vi "Impedance_Multi_WrapSingle.vi"() -> ()   [LabVIEW 2021]
uses:
  <vilib>/Analysis/1siggen.llb/Ramp Pattern by Samples.vi
  <vilib>/Analysis/baseanly.llb/Mean (DBL).vi
  <vilib>/Analysis/NI_AALBase.lvlib
panel:
  out "Test Number":i32
  in  "Num Avg":i32=5
  out "Mean Phase":dbl format="%0.2f"
  out "Mean Mag":dbl format="%.4p"
  out "Phase Graph":cluster{dbl[], "Ramp Pattern":dbl[]}(graph)
  in  "amplitude":dbl=0.1 format="%0.2p"
  in  "SampRate":dbl=250000.0 format="%0.2f"
  in  "Test Time":dbl=1.0 format="%#_6p"
  out "Mag Graph":cluster{dbl[], "Ramp Pattern":dbl[]}(graph)
  in  "samples":i32=128
  in  "start":dbl format="%#.4p"
  in  "end freq":dbl=1.0 format="%#.4p"
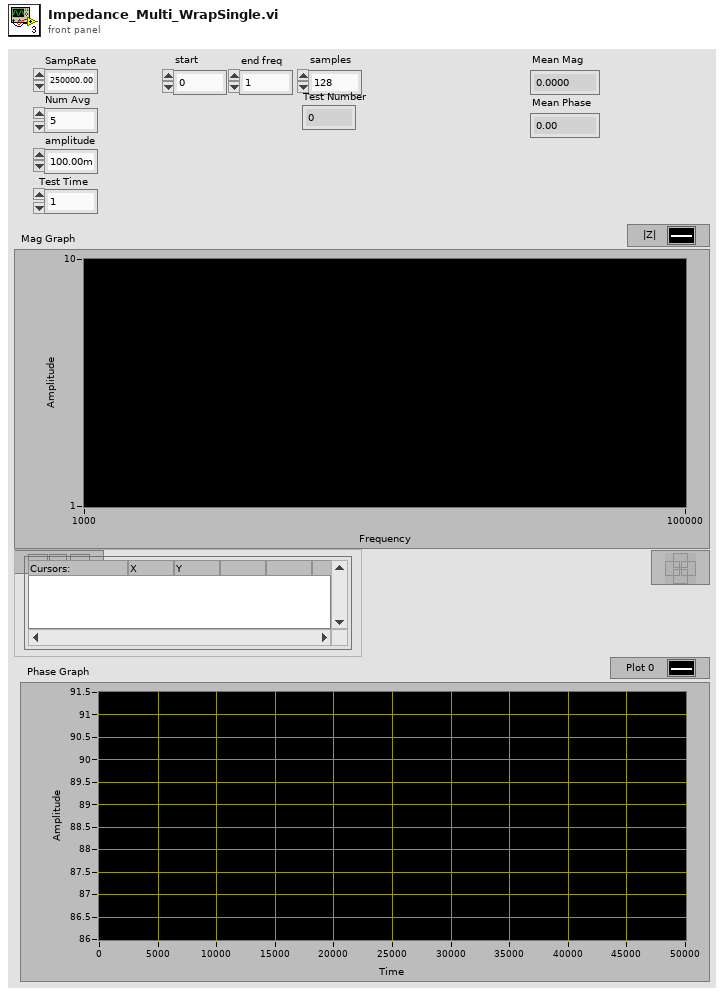
[diagram p1: front panel]
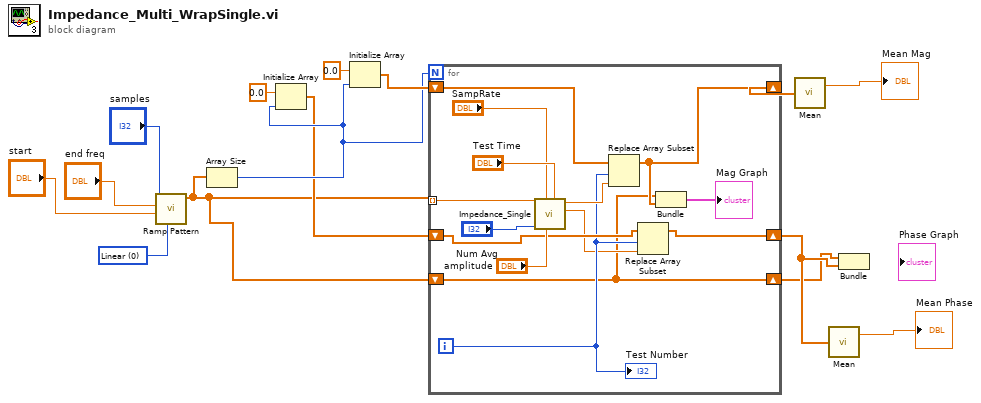
[diagram p0: block diagram]
diagram:
  w12 = u16 0 items=["Linear", "Logarithmic"] ("type")
  n1 = call-poly <vilib>:"Ramp Pattern.vi"("type"=w12, "start"="start", "end"="end freq", "samples"="samples") -> ("Ramp Pattern"=w3:dbl[])  [unwired: 6 in, 1 out]
  n2 = Array Size(array=w3) -> (size(s)=w8:i32)
  n3 = Initialize Array(0.0 ("element"), w8) -> (w7:dbl[])
  n4 = Initialize Array(0.0 ("element"), w8) -> (w10:dbl[])
  n5 = for {
    N: w8 -> [_]
    tunnel: w3 -> [w29] mode=indexing
    shift-right: [w17] -> w6
    shift-left: w10 -> [w28]
    shift-right: [w19] -> w2
    shift-left: w7 -> [w25]
    shift-right: [w16] -> w1
    shift-left: w3 -> [w16]
    i -> [w24]
    n6 = call "Impedance_Single.vi"("Sampling Time"="Test Time", "Amplitude (pk)"="amplitude", "Sampling Rate"="SampRate", "Number of runs"="Num Avg", "Measure Frequency"=w29) -> ("Impedance (Phase)"=w23:dbl, "Impedance (Mag)"=w27:dbl)  [unwired: 4 in]
    n7 = Replace Array Subset(array=w28, new element=w27, index=w24) -> (w17:dbl[])
    n8 = Replace Array Subset(array=w25, new element=w23, index=w24) -> (w19:dbl[])
    n9 = Bundle("Ramp Pattern"=w16, w17) -> (→"Mag Graph":cluster{"Ramp Pattern":dbl[], dbl[]})  [unwired: 1 in]
    "Test Number" <- w24
  }
  n10 = call-poly <vilib>:"Mean.vi"("X"=w6) -> ("mean"=→"Mean Mag":dbl)  [unwired: 1 out]
  n11 = call-poly <vilib>:"Mean.vi"("X"=w2) -> ("mean"=→"Mean Phase":dbl)  [unwired: 1 out]
  n12 = Bundle("Ramp Pattern"=w1, w2) -> ()  [unwired: 1 in, 1 out]
